vi "Size Table.vi"(8 "error in (no error)":errorcluster, 10 "Table":refnum<vi>, 11 "Tab Control":refnum<vi>) -> (0 "error out":errorcluster)   [LabVIEW 2016, in "System Mapping Tool.lvlib"]
uses:
  System Mapping Tool.lvlib
  <vilib>/Utility/miscctls.llb/LVRowAndColumnTypeDef.ctl
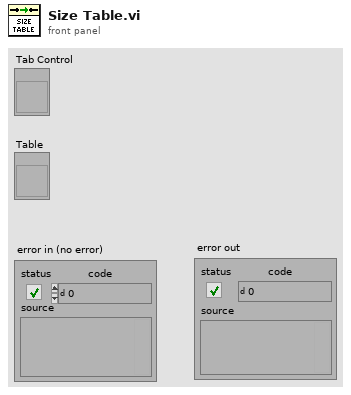
[diagram p1: front panel]
types:
  T1 = typedef "LVRowAndColumnTypeDef.ctl" = cluster{"Row":i32, "Column":i32}
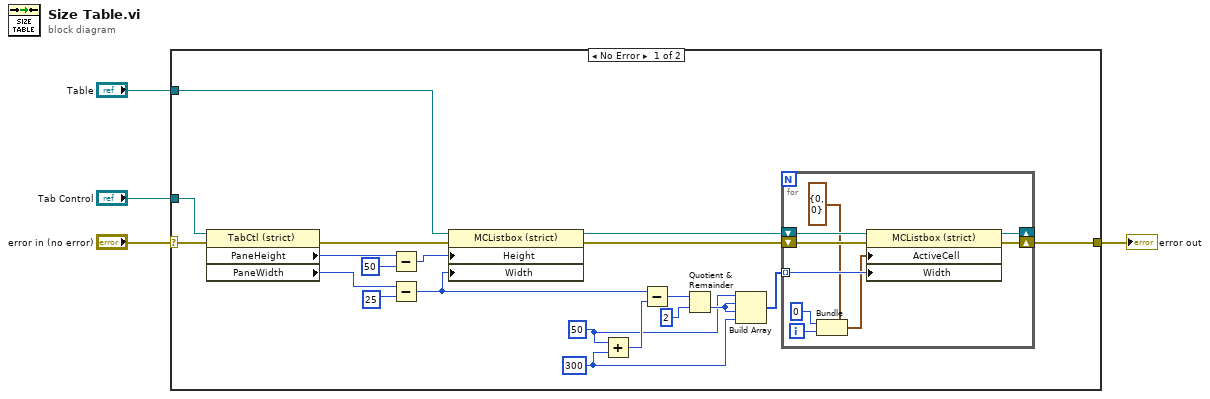
[diagram p0: block diagram]
diagram:
  n1 = case shown="No Error" "error in (no error)" {
    selector: "error in (no error)" -> [w24 w34]
    tunnel: [w5 w34] -> w3
    tunnel: "Tab Control" -> [w23 _]
    tunnel: "Table" -> [w22 _]
    frame No Error {
      w15 = u32 300 ("Bounds:Area Width")
      w10 = u32 50 ("Bounds:Area Width")
      n2 = property class="TabCtl (strict)"(reference=w23, error in=w24) -> (error out=w21:errorcluster, "PaneHeight"=w20:u32, "PaneWidth"=w17:u32)  [unwired: 1 out]
      n3 = Subtract(x=w20, y=u32 50) -> (x-y=w18:u32)
      n4 = Subtract(x=w17, y=u32 25) -> (x-y=w12:u32)
      n5 = property class="MCListbox (strict)"(reference=w22, error in=w21, "Height"=w18, "Width"=w12) -> (reference out=w7:refnum<vi>, error out=w8:errorcluster)
      n6 = Add(x=w10, y=w15) -> (x+y=w11:u32)
      n7 = Subtract(x=w12, y=w11) -> (x-y=w9:u32)
      n8 = Quotient & Remainder(x=w9, y=u32 2) -> (floor(x/y)=w14:u32)  [unwired: 1 out]
      n9 = Build Array(w10, w14, w14, w15) -> (w6:u32[])
      n10 = for {
        shift-right: [w31] -> _
        shift-left: w7 -> [w33]
        shift-right: [w30] -> w5
        shift-left: w8 -> [w32]
        tunnel: w6 -> [w29] mode=indexing
        i -> [w28]
        n11 = Bundle(cluster=T1 {"Row"=0, "Column"=0} ("Active Cell:Active Cell"), "Row"=0, "Column"=w28) -> (w26:T1)
        n12 = property class="MCListbox (strict)"(reference=w33, error in=w32, "ActiveCell"=w26, "Width"=w29) -> (reference out=w31:refnum<vi>, error out=w30:errorcluster)
      }
    }
    frame Error {
    }
  }
  "error out" <- w3
